vi "GitFetch.vi"(8 "error in (no error)":errorcluster, 11 "Directory (leave empty for relative)":path) -> (0 "error out":errorcluster, 3 "directory out":path=path "C:/RageATE/Labview Utilities/GitTools", 5 "Git Ok?(t)":bool)   [LabVIEW 2018]
panel:
  out "standard output 2":string
  out "standard error":string="POST git-upload-pack (154 bytes)\nFrom https://github.com/RaGESystemsCGH/RageATE\n   e4d4f6d6..d921aa86  main       -> origin/main\n"
  out "standard output":string="!!!SW is not up to date with origin on server.\nCheck the message and correct the issue using Github!!\n\n\nPOST git-upload-pack (154 bytes)\nFrom https://github.com/RaGESystemsCGH/RageATE\n   e4d4f6d6..d921aa86  main       -> origin/main\n"
  out "git status":string[](array[string])=["POST git-upload-pack (154 bytes)", "From https://github.com/RaGESystemsCGH/RageATE", "   e4d4f6d6..d921aa86  main       -> origin/main"]
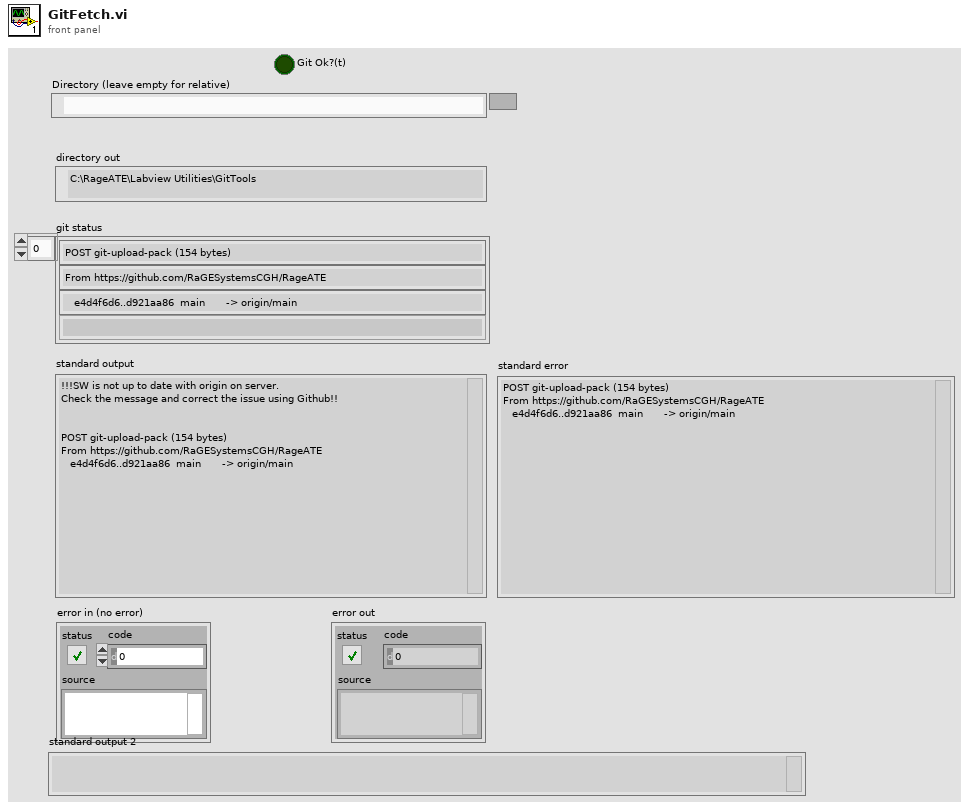
[diagram p1: front panel]
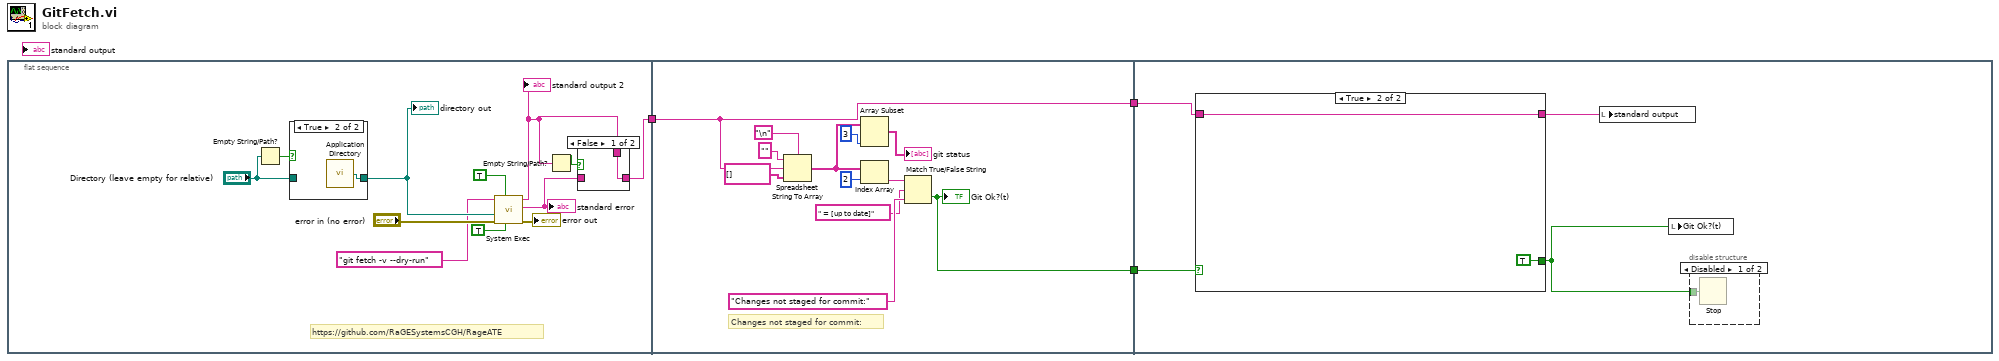
[diagram p0: block diagram]
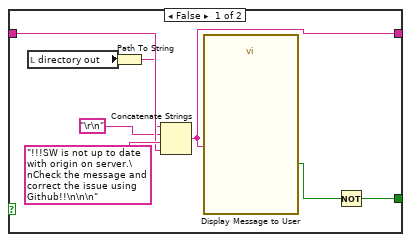
[diagram p5: hidden frame]
diagram:
  n1 = flat-sequence {
    tunnel: [w6] -> w2
    tunnel: [w21] -> w3
    tunnel: w2 -> [w20]
    tunnel: [w20] -> w1
    tunnel: w3 -> [w35]
    tunnel: w1 -> [w34]
    frame #0 {
      # "https://github.com/RaGESystemsCGH/RageATE"
      n2 = Empty String/Path?(string/path="Directory (leave empty for relative)") -> (empty?=w10:bool)
      n3 = case shown="True" w10 {
        tunnel: [w18 w19] -> w12
        tunnel: "Directory (leave empty for relative)" -> [w18 _]
        frame False {
        }
        frame True {
          n4 = call <vilib>:"Application Directory.vi"() -> ("Application Directory"=w19:path)
        }
      }
      "directory out" <- w12
      n5 = call <vilib>:"System Exec.vi"("run minimized? (F)"=TRUE, "wait until completion? (T)"=TRUE, "error in (no error)"="error in (no error)", "working directory"=w12, "command line"="git fetch -v --dry-run") -> ("error out"=→"error out":errorcluster, "standard error"=w5:string, "standard output"=w4:string)  [unwired: 3 in, 1 out]
      "standard error" <- w5
      "standard output 2" <- w4
      n6 = Empty String/Path?(string/path=w4) -> (empty?=w7:bool)
      n7 = case shown="False" w7 {
        tunnel: [w16 w17] -> w6
        tunnel: w5 -> [_ w17]
        tunnel: w4 -> [w16 _]
        frame False {
        }
        frame True {
        }
      }
    }
    frame #1 {
      # "Changes not staged for commit:"
      n8 = Spreadsheet String To Array(delimiter (Tab)="\n", format string="", spreadsheet string=w20, array type (2D Dbl)=string[] []) -> (array=w30:string[])
      n9 = Array Subset(array=w30, length=3) -> (→"git status":string[])  [unwired: 1 in]
      n10 = Index Array(array=w30, index=2) -> (element=w31:string)
      n11 = Match True/False String(2:"Changes not staged for commit:" ("false string"), 3:" = [up to date]" ("false string"), 4:w31) -> (0:w21:bool)  [unwired: 1 out]
      "Git Ok?(t)" <- w21
    }
    frame #2 {
      n12 = case shown="True" w35 {
        tunnel: [w42 w46] -> w33
        tunnel: w34 -> [w43 w46]
        tunnel: [w37 TRUE ("STOP")] -> w32
        frame False {
          n13 = local read "directory out"() -> (w40:path)
          n14 = Path To String(path=w40) -> (string=w39:string)
          n15 = Concatenate Strings(w39, "\r\n", "!!!SW is not up to date with origin on server.\nCheck the message and correct the issue using Github!!\n\n\n", w43) -> (w42:string)
          n16 = call "Display Message to User"("Message"=w42) -> ("STOP"=w41:bool)  [unwired: 9 in, 1 out]
          n17 = Not(x=w41) -> (.not. x?=w37:bool)
        }
        frame True {
        }
      }
      n18 = local write "standard output"(w33) -> ()
      n19 = local write "Git Ok?(t)"(w32) -> ()
      n20 = disable-structure shown="Disabled" {
        disable-tunnel: w32 -> [w36 _]
        frame Disabled {
          n21 = Stop(stop? (T)=w36) -> ()
        }
        frame Enabled {
        }
      }
    }
  }
